vi "something vs T.vi"() -> ()   [LabVIEW 2016]
uses:
  subs/path list.vi
  <vilib>/Analysis/NI_AALPro.lvlib
panel:
  in  "B value":dbl format="%.4f"
  in  "save plots?":bool
  in  "format":string="%.6e"
  in  "temperatures":dbl[](array[numeric]) format="%.4f"
  out "plotted data":cluster{"temperatures":dbl[], dbl[]}(graph)
  in  "type of interpolation":u16(ring) items=["linear", "cubic spline", "polynomial"]
  in  "y domain":u16(ring) items=["channel A"]
  in  "x domain":u16(ring) items=["B (rising field)", "B (falling field)"]
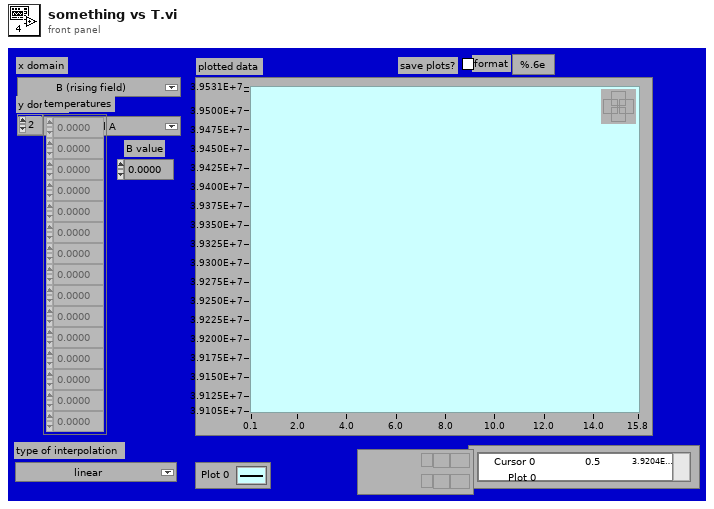
[diagram p1: front panel]
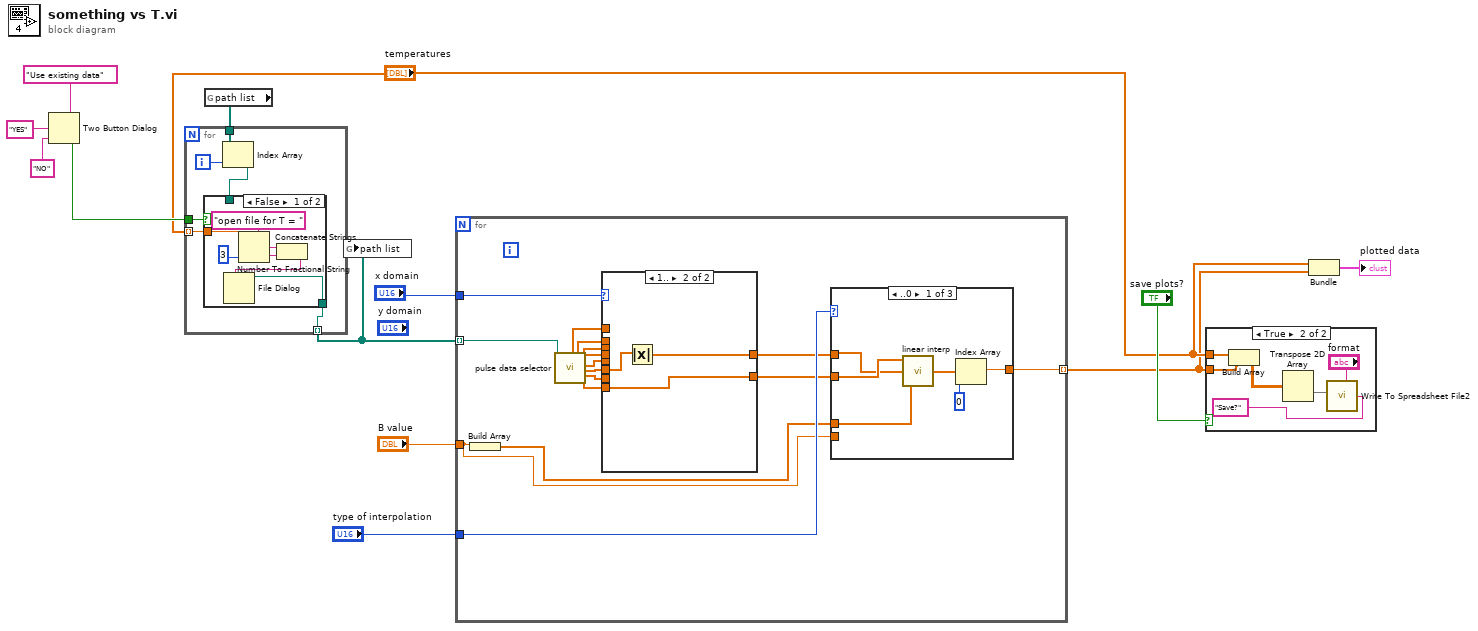
[diagram p0: block diagram]
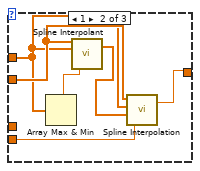
[diagram p4: hidden frame]
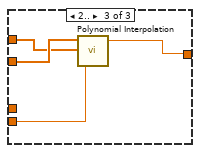
[diagram p5: hidden frame]
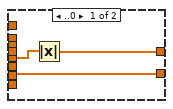
[diagram p6: hidden frame]
diagram:
  n1 = Two Button Dialog(message="Use existing data", 1:"NO", 2:"YES") -> (T button?=w6:bool)
  n2 = global read "path list.vi" "path list"() -> (w10:path[])
  n3 = for {
    tunnel: "temperatures" -> [w19] mode=indexing
    tunnel: [w18] -> w11 mode=indexing
    tunnel: w10 -> [w16]
    tunnel: w6 -> [w17]
    i -> [w15]
    n4 = Index Array(array=w16, index=w15) -> (element=w14:path)
    n5 = case shown="False" w17 {
      tunnel: w19 -> [w21 _]
      tunnel: [w20 w26] -> w18
      tunnel: w14 -> [_ w26]
      frame False {
        n6 = Number To Fractional String(number=w21, precision (6)=3) -> (F-format string=w24:string)  [unwired: 2 in]
        n7 = Concatenate Strings("open file for T = ", w24) -> (w25:string)
        n8 = File Dialog(7:w25) -> (3:w20:path)  [unwired: 6 in, 3 out]
      }
      frame True {
      }
    }
  }
  n9 = global write "path list.vi" "path list"(w11) -> ()
  n10 = for {
    tunnel: "x domain" -> [w34]
    tunnel: "type of interpolation" -> [w32]
    tunnel: w11 -> [w33] mode=indexing
    tunnel: "B value" -> [w28]
    tunnel: [w27] -> w2 mode=indexing
    n11 = Build Array(w28) -> (w31:dbl[])
    n12 = call "pulse data selector.vi"("file path (dialog if empty)"=w33) -> ("time rising"=w37:dbl[], "time falling"=w38:dbl[], "dB/dt rising"=w36:dbl[], "dB/dt falling"=w35:dbl[], "B rising"=w41:dbl[], "B falling"=w42:dbl[], "ch A rising"=w39:dbl[], "ch A falling"=w40:dbl[])  [unwired: 6 in, 5 out]
    n13 = case shown="1.." w34 {
      tunnel: w37 -> [_ _]
      tunnel: w38 -> [_ _]
      tunnel: w39 -> [w60 _]
      tunnel: w40 -> [_ w62]
      tunnel: w41 -> [w61 _]
      tunnel: w42 -> [_ w64]
      tunnel: w36 -> [_ _]
      tunnel: w35 -> [_ _]
      tunnel: [w60 w62] -> w29
      tunnel: [w59 w63] -> w30
      frame ..0 {
        n14 = Absolute Value(x=w61) -> (abs(x)=w59:dbl[])
      }
      frame 1.. {
        n15 = Absolute Value(x=w64) -> (abs(x)=w63:dbl[])
      }
    }
    n16 = case shown="..0" w32 {
      tunnel: w31 -> [w46 _ _]
      tunnel: w30 -> [w47 w51 w57]
      tunnel: w29 -> [w48 w52 w58]
      tunnel: [w43 w49 w55] -> w27
      tunnel: w28 -> [_ w50 w56]
      frame ..0 {
        n17 = call "linear interp.vi"("x array"=w46, "X data"=w47, "Y data"=w48) -> ("y"=w44:dbl[])
        n18 = Index Array(array=w44, index=0) -> (element=w43:dbl)
      }
      frame 1 {
        n19 = Array Max & Min(array=w51) -> (max value=w54:dbl)  [unwired: 3 out]
        n20 = call <vilib>:"Spline Interpolant.vi"("final boundary"=w54, "X"=w51, "Y"=w52) -> ("Interpolant"=w53:dbl[])  [unwired: 1 in, 1 out]
        n21 = call <vilib>:"Spline Interpolation.vi"("x value"=w50, "Interpolant"=w53, "X"=w51, "Y"=w52) -> ("interpolation value"=w49:dbl)  [unwired: 1 out]
      }
      frame 2.. {
        n22 = call <vilib>:"Polynomial Interpolation.vi"("x value"=w56, "X"=w57, "Y"=w58) -> ("interpolation value"=w55:dbl)  [unwired: 2 out]
      }
    }
  }
  n23 = case shown="True" "save plots?" {
    tunnel: w2 -> [_ w69]
    tunnel: "temperatures" -> [_ w66]
    frame False {
    }
    frame True {
      n24 = Build Array(w66, w69) -> (w67:dbl[][])
      n25 = Transpose 2D Array(2D array=w67) -> (transposed array=w68:dbl[][])
      n26 = call "Write To Spreadsheet File2.vi"("dialogue"="Save?", "format (%.3f)"="format", "2D data"=w68) -> ()  [unwired: 5 in, 1 out]
    }
  }
  n27 = Bundle("temperatures"="temperatures", w2) -> (→"plotted data":cluster{"temperatures":dbl[], dbl[]})  [unwired: 1 in]
